vi "ResetTrigger.vi"(8 "error in":errorcluster, 11 "TriggerBox in":refnum<class "TriggerBox.lvclass">) -> (0 "error out":errorcluster, 3 "TriggerBox out":refnum<class "TriggerBox.lvclass">)   [LabVIEW 2013, in "TriggerBox.lvclass"]
uses:
  TriggerBox.lvclass
  <vilib>/Utility/error.llb/Error Cluster From Error Code.vi
  <vilib>/rvi/errors/niLvFpgaAdjustHostInterfaceError.vi
  RT/FPGASession/FPGARef.ctl
  <vilib>/rvi/interface/nirviReadWriteControl/nirviReadWriteControl.xnode
  FPGA Bitfiles/HWSWTriggerBox_FPGATarget2_TriggerBox_1zhzIx5zPP8.lvbitx
  FPGAMain.vi
  FPGASessionClass/FPGASession.lvclass
  NiFpgaLv.dll
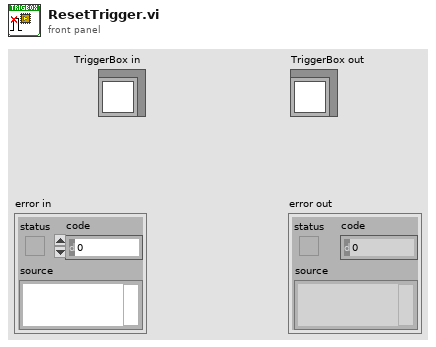
[diagram p1: front panel]
types:
  T1 = typedef "FPGASession.lvclass/FPGARef.ctl" = refnum<k20>
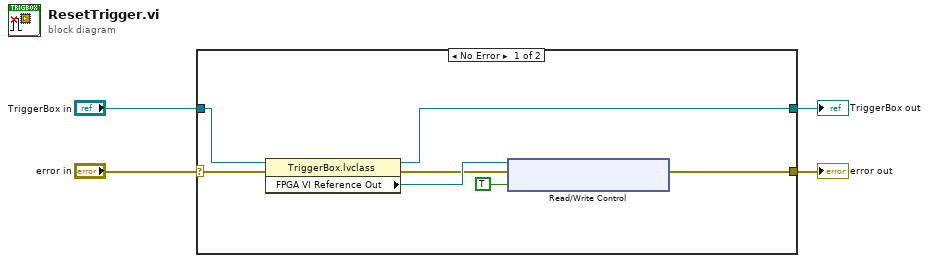
[diagram p0: block diagram]
diagram:
  n1 = case shown="No Error" "error in" {
    selector: "error in" -> [w8 w13]
    tunnel: [w11 w13] -> w1
    tunnel: [w5 w12] -> w2
    tunnel: "TriggerBox in" -> [w7 w12]
    frame No Error {
      n2 = property class="TriggerBox.lvclass"(reference=w7, error in=w8) -> (reference out=w5:refnum<class "TriggerBox.lvclass">, error out=w6:errorcluster, "FPGA VI Reference Out"=w9:T1)
      n3 = xnode "Read/Write Control"("FPGA VI Reference In"=w9, "error in"=w6, "ResetTrigger"=TRUE) -> ("error out"=w11:errorcluster)  [unwired: 1 out]
    }
    frame Error {
    }
  }
  "error out" <- w1
  "TriggerBox out" <- w2
